vi "Write to Instrument.vi"(7 "Slave Address":i32=-1 min=-1 max=30 step=1, 8 "error":errorcluster, 10 "Command":string, 11 "VISA":refnum<visa-resource-name>) -> (0 "error out":errorcluster, 3 "VISA out":refnum<visa-resource-name>)   [LabVIEW 2019, in "TDK-Lambda GEN LAN Series.lvlib"]
doc: "Sends any SCPI command to the GEN power supply \n\nIf the command returns an error (from the instrument's SYST:ERR queue), the VI path, command string and SYST:ERR message are sent to the \"error out\" string."
uses:
  <instrlib>/TDK-Lambda GEN LAN Series/TDK-Lambda GEN LAN Series.lvlib
panel:
  # "TDK-Lambda Genesys \n LAN\n  DC Power Supplies"
  # "Send Any Command"
  # "After command sent, \nsystem error is checked"
  # "(c) 2019 TDK-Lambda.  ALL RIGHTS RESERVED."
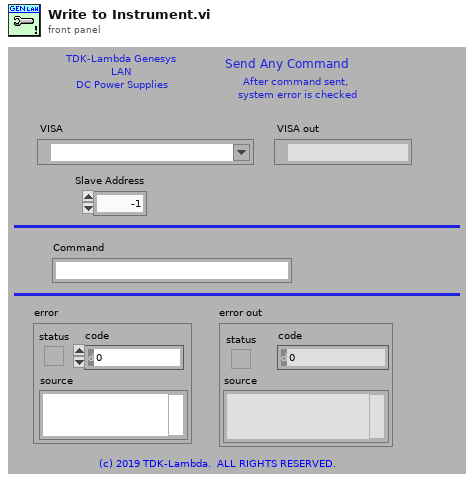
[diagram p1: front panel]
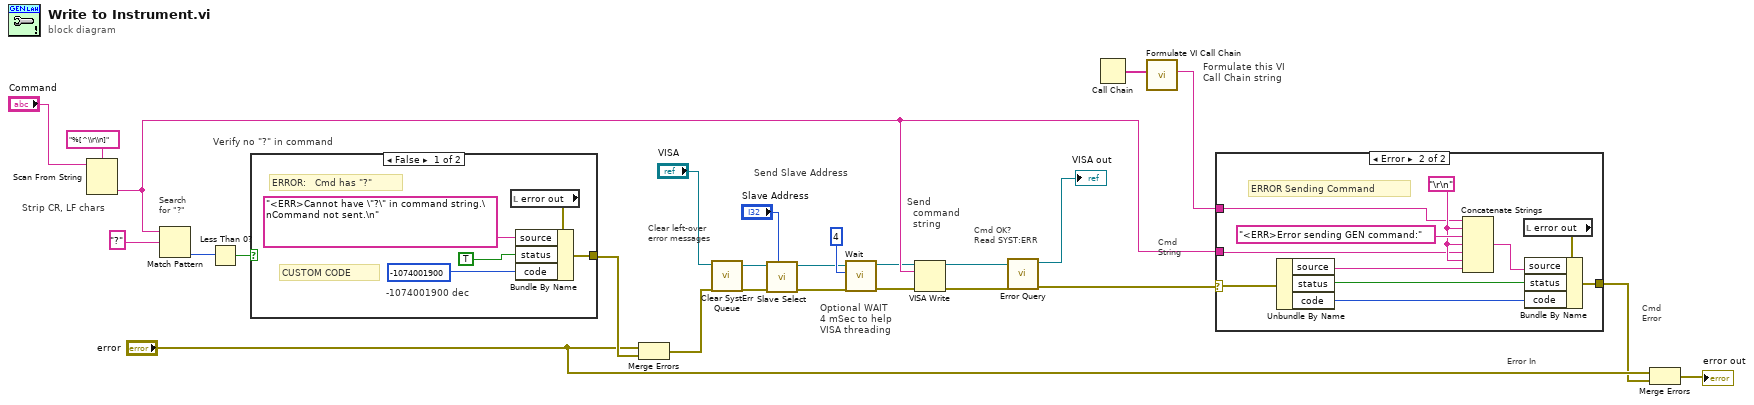
[diagram p0: block diagram]
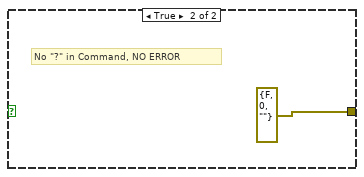
[diagram p2: hidden frame]
diagram:
  # "Optional WAIT \n4 mSec to help \nVISA threading"
  # "Cmd OK?\nRead SYST:ERR"
  # "Send Slave Address"
  # "Cmd\nError"
  # "Error In"
  # "Cmd\nString"
  # "Verify no \"?\" in command"
  # "Clear left-over \nerror messages"
  # "Send  \n  command  \n  string"
  # "Search\nfor \"?\""
  # "Strip CR, LF chars"
  # "Formulate this VI \nCall Chain string"
  n1 = Scan From String(format string="%[^\\r\\n]", input string="Command") -> (output 1=w16:string)  [unwired: 3 in, 3 out]
  n2 = Match Pattern(string=w16, regular expression="?") -> (offset past match=w23:i32)  [unwired: 1 in, 3 out]
  n3 = Less Than 0?(x=w23) -> (x < 0?=w24:bool)
  n4 = case shown="False" w24 {
    tunnel: [w28 errorcluster {"status"=FALSE, "code"=0, "source"=""} ("error out")] -> w21
    frame False {
      # "-1074001900 dec"
      # "CUSTOM CODE"
      # "ERROR:   Cmd has \"?\""
      n5 = local read "error out"() -> (w31:errorcluster)
      n6 = Bundle By Name(cluster=w31, "source"="<ERR>Cannot have \"?\" in command string.\nCommand not sent.\n" ("Source"), "status"=TRUE, "code"=-1074001900) -> (w28:errorcluster)
    }
    frame True {
      # "No \"?\" in Command, NO ERROR"
    }
  }
  n7 = Merge Errors("error", w21) -> (w20:errorcluster)
  n8 = call <instrlib>:"Clear SystErr Queue.vi"("error"=w20, "VISA"="VISA") -> ("error out"=w9:errorcluster, "VISA out"=w10:refnum<visa-resource-name>)  [unwired: 8 in]
  n9 = call <instrlib>:"Slave Select.vi"("Slave Address"="Slave Address", "error"=w9, "VISA"=w10) -> ("error out"=w4:errorcluster, "VISA out"=w5:refnum<visa-resource-name>)  [unwired: 7 in]
  n10 = call <instrlib>:"Wait.vi"("error"=w4, "Delay (20 mS)"=u32 4, "VISA"=w5) -> ("error out"=w2:errorcluster, "VISA out"=w3:refnum<visa-resource-name>)  [unwired: 7 in]
  n11 = VISA Write(VISA resource name=w3, write buffer=w16, error in (no error)=w2) -> (VISA resource name out=w8:refnum<visa-resource-name>, error out=w7:errorcluster)  [unwired: 1 out]
  n12 = call <instrlib>:"Error Query.vi"("error"=w7, "VISA"=w8) -> ("error out"=w18:errorcluster, "VISA out"=→"VISA out":refnum<visa-resource-name>)  [unwired: 6 in, 2 out]
  n13 = Call Chain() -> (call chain=w12:string[])
  n14 = call <instrlib>:"Formulate VI Call Chain.vi"("Call Chain"=w12) -> ("String Out"=w11:string)  [unwired: 10 in]
  n15 = case shown="Error" w18 {
    selector: w18 -> [w33 w39]
    tunnel: w16 -> [_ w40]
    tunnel: [w33 w35] -> w14
    tunnel: w11 -> [_ w34]
    frame No Error {
      # "Command Sent Correctly \n  and No \"SYST:ERR?\" Returned"
    }
    frame Error {
      w41 = "\r\n"
      # "ERROR Sending Command"
      n16 = Unbundle By Name(w39) -> ("source"=w36:string, "status"=w37:bool, "code"=w38:i32)
      n17 = Concatenate Strings(w34, w41, "<ERR>Error sending GEN command:" ("Source"), w41, w40, w41, w36) -> (w43:string)
      n18 = local read "error out"() -> (w44:errorcluster)
      n19 = Bundle By Name(cluster=w44, "source"=w43, "status"=w37, "code"=w38) -> (w35:errorcluster)
    }
  }
  n20 = Merge Errors("error", w14) -> (→"error out":errorcluster)
